vi "SINGLE Measurement.vi"(1 "VISA resource name":refnum<visa-resource-name>="GPIB12::28::INSTR") -> (2 "Vexc":dbl=nan format="%.8f", 3 "loss":dbl=nan format="%.8f", 4 "capacitance":dbl=nan format="%.8f")   [LabVIEW 2016]
panel:
  in  "byte count":u32=128
  out "read buffer":string
  out "error out":errorcluster={"status"=TRUE, "code"=-1073807195, "source"="VISA Write in command send.vi"} {"code" format="%.0x"}
  in  "error in":errorcluster {"code" format="%.0x"}
  # "Do a single measurement"
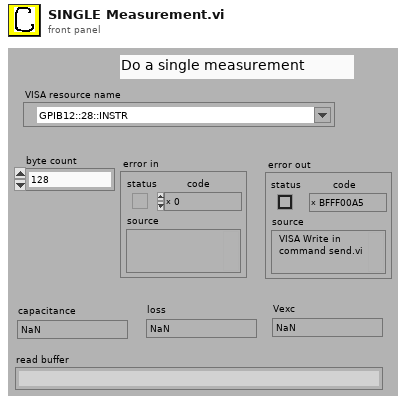
[diagram p1: front panel]
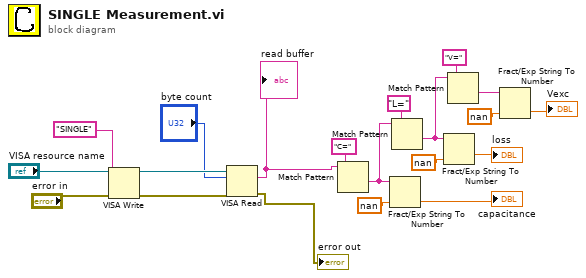
[diagram p0: block diagram]
diagram:
  n1 = VISA Write(VISA resource name="VISA resource name", write buffer="SINGLE", error in (no error)="error in") -> (VISA resource name out=w18:refnum<visa-resource-name>, error out=w17:errorcluster)  [unwired: 1 out]
  n2 = VISA Read(VISA resource name=w18, byte count="byte count", error in (no error)=w17) -> (read buffer=w2:string, error out=→"error out":errorcluster)  [unwired: 2 out]
  "read buffer" <- w2
  n3 = Match Pattern(string=w2, regular expression="C=") -> (after substring=w9:string)  [unwired: 1 in, 3 out]
  n4 = Fract/Exp String To Number(string=w9, default (0 dbl)=nan) -> (number=→"capacitance":dbl)  [unwired: 2 in, 1 out]
  n5 = Match Pattern(string=w9, regular expression="L=") -> (after substring=w4:string)  [unwired: 1 in, 3 out]
  n6 = Fract/Exp String To Number(string=w4, default (0 dbl)=nan) -> (number=→"loss":dbl)  [unwired: 2 in, 1 out]
  n7 = Match Pattern(string=w4, regular expression="V=") -> (after substring=w7:string)  [unwired: 1 in, 3 out]
  n8 = Fract/Exp String To Number(string=w7, default (0 dbl)=nan) -> (number=→"Vexc":dbl)  [unwired: 2 in, 1 out]
